vi "Convert String to Typed Value.vi"(8 "error in":errorcluster, 10 "Value":string, 11 "DataType":u16(ring) items=["UNKNOWN", "BOOLEAN", "INTEGER8", "INTEGER16", "INTEGER32", "UNSIGNED8", "UNSIGNED16", "UNSIGNED32", "REAL32", "VISIBLE_STRING", "OCTET_STRING", "UNICODE_STRING", "TIME_OF_DAY", "TIME_DIFFERENCE", "RESERVED1", "DOMAIN", "INTEGER24", "REAL64", "INTEGER40", "INTEGER48", "INTEGER56", "INTEGER64", "UNSIGNED24", "RESERVED2", "UNSIGNED40", "UNSIGNED48", "UNSIGNED56", "UNSIGNED64", "RESERVED3", "RESERVED4", "RESERVED5", "RESERVED6", "PDO_COMMUNICATION_PARAMETER", "PDO_MAPPING", "SDO_PARAMETER", "IDENTITY", "RESERVED7"]) -> (0 "error out":errorcluster, 3 "Typed Value":variant)   [LabVIEW 2020, in "CANopen.lvlib"]
uses:
  CANopen.lvlib
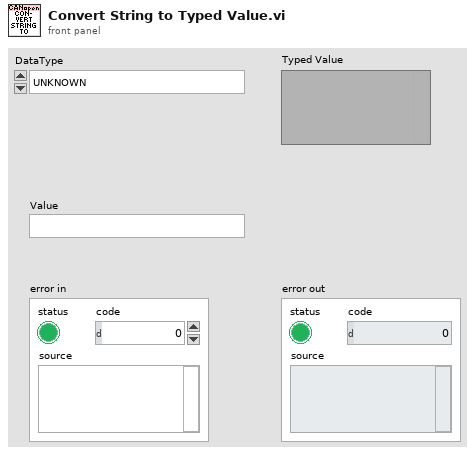
[diagram p1: front panel]
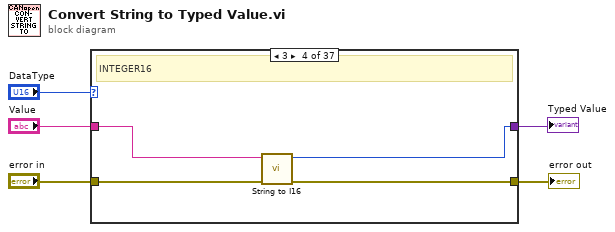
[diagram p0: block diagram]
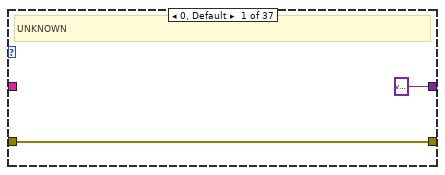
[diagram p2: hidden frame]
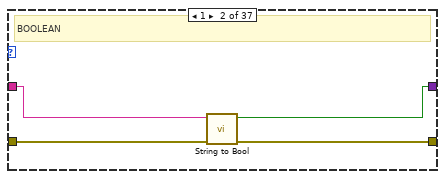
[diagram p3: hidden frame]
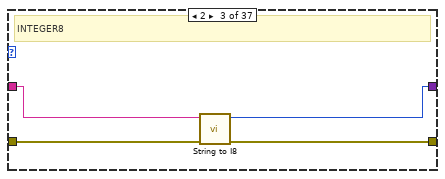
[diagram p4: hidden frame]
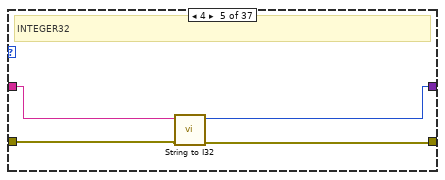
[diagram p5: hidden frame]
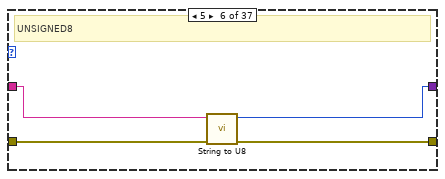
[diagram p6: hidden frame]
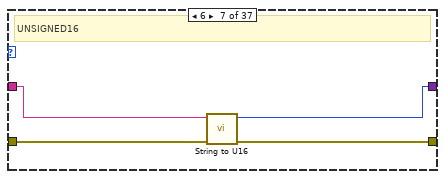
[diagram p7: hidden frame]
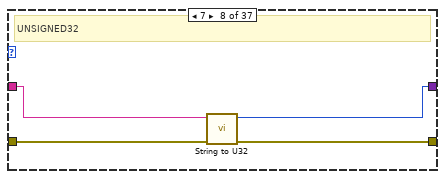
[diagram p8: hidden frame]
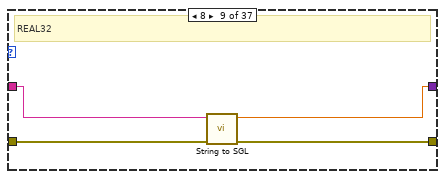
[diagram p9: hidden frame]
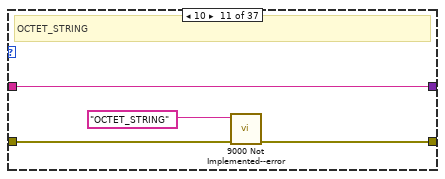
[diagram p11: hidden frame]
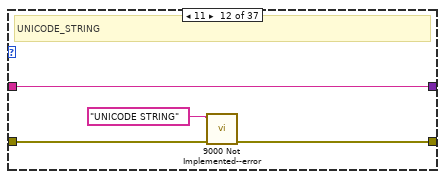
[diagram p12: hidden frame]
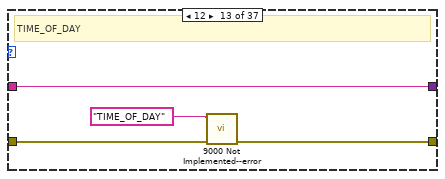
[diagram p13: hidden frame]
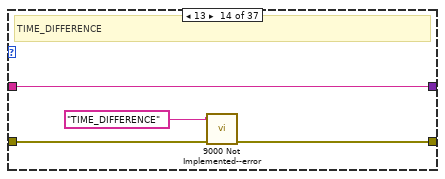
[diagram p14: hidden frame]
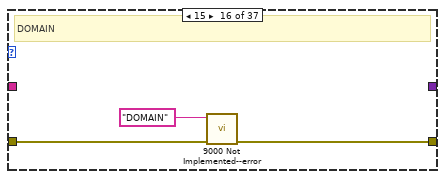
[diagram p16: hidden frame]
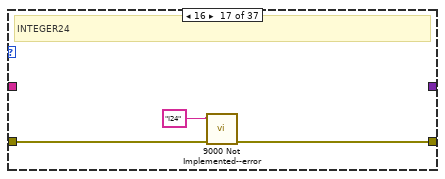
[diagram p17: hidden frame]
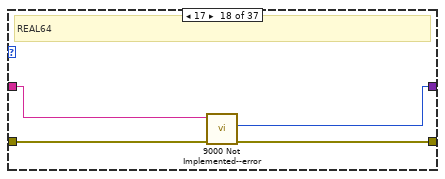
[diagram p18: hidden frame]
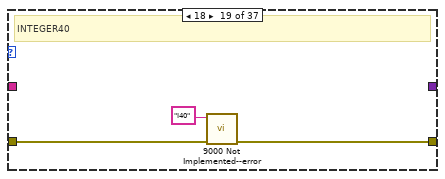
[diagram p19: hidden frame]
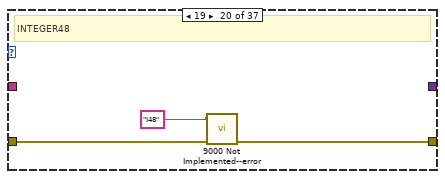
[diagram p20: hidden frame]
diagram:
  n1 = case shown="3" "DataType" {
    tunnel: [variant w8 w12 w16 w20 w24 w28 w32 w36 w41 w45 w48 w52 w57 _ _ _ w65 _ _ _ _ _ _ _ _ _ w94 _ _ _ _ _ _ _ _ _] -> w4
    tunnel: "error in" -> [w7 w11 w15 w19 w23 w27 w31 w35 w39 w40 w44 w49 w53 w56 w58 w61 w64 w68 w71 w74 w77 w80 w83 w84 w87 w90 w93 w97 w98 w99 w100 w101 w104 w107 w110 w113 w114]
    tunnel: [w7 w10 w13 w18 w22 w26 w30 w34 w38 w40 w43 w47 w51 w55 w58 w60 w63 w67 w70 w73 w76 w79 w82 w84 w86 w89 w92 w96 w98 w99 w100 w101 w103 w106 w109 w112 w114] -> w3
    tunnel: "Value" -> [_ w9 w14 w17 w21 w25 w29 w33 w37 w41 w45 w48 w52 w57 _ _ _ w66 _ _ _ w78 _ _ _ _ _ w95 _ _ _ _ _ _ _ _ _]
    frame 0, Default {
      # "UNKNOWN"
    }
    frame 1 {
      # "BOOLEAN"
      n2 = call "String to Bool.vi"("error in"=w11, "Integer String"=w9) -> ("error out"=w10:errorcluster, "Bool"=w8:bool)  [unwired: 8 in]
    }
    frame 2 {
      # "INTEGER8"
      n3 = call "String to I8.vi"("error in"=w15, "Integer String"=w14) -> ("error out"=w13:errorcluster, "I8"=w12:i8)  [unwired: 8 in]
    }
    frame 3 {
      # "INTEGER16"
      n4 = call "String to I16.vi"("error in"=w19, "Integer String"=w17) -> ("error out"=w18:errorcluster, "I16"=w16:i16)  [unwired: 8 in]
    }
    frame 4 {
      # "INTEGER32"
      n5 = call "String to I32.vi"("error in"=w23, "Integer String"=w21) -> ("error out"=w22:errorcluster, "I32"=w20:i32)  [unwired: 8 in]
    }
    frame 5 {
      # "UNSIGNED8"
      n6 = call "String to U8.vi"("error in"=w27, "Integer String"=w25) -> ("error out"=w26:errorcluster, "U8"=w24:u8)  [unwired: 8 in]
    }
    frame 6 {
      # "UNSIGNED16"
      n7 = call "String to U16.vi"("error in"=w31, "Integer String"=w29) -> ("error out"=w30:errorcluster, "U16"=w28:u16)  [unwired: 8 in]
    }
    frame 7 {
      # "UNSIGNED32"
      n8 = call "String to U32.vi"("error in"=w35, "Integer String"=w33) -> ("error out"=w34:errorcluster, "U32"=w32:u32)  [unwired: 8 in]
    }
    frame 8 {
      # "REAL32"
      n9 = call "String to SGL.vi"("error in"=w39, "Integer String"=w37) -> ("error out"=w38:errorcluster, "SGL"=w36:sgl)  [unwired: 8 in]
    }
    frame 9 {
      # "VISIBLE_STRING"
    }
    frame 10 {
      # "OCTET_STRING"
      n10 = call "9000 Not Implemented--error.vi"("error in"=w44, "Argument"="OCTET_STRING") -> ("error out"=w43:errorcluster)  [unwired: 8 in, 1 out]
    }
    frame 11 {
      # "UNICODE_STRING"
      n11 = call "9000 Not Implemented--error.vi"("error in"=w49, "Argument"="UNICODE STRING") -> ("error out"=w47:errorcluster)  [unwired: 8 in, 1 out]
    }
    frame 12 {
      # "TIME_OF_DAY"
      n12 = call "9000 Not Implemented--error.vi"("error in"=w53, "Argument"="TIME_OF_DAY") -> ("error out"=w51:errorcluster)  [unwired: 8 in, 1 out]
    }
    frame 13 {
      # "TIME_DIFFERENCE"
      n13 = call "9000 Not Implemented--error.vi"("error in"=w56, "Argument"="TIME_DIFFERENCE") -> ("error out"=w55:errorcluster)  [unwired: 8 in, 1 out]
    }
    frame 14 {
      # "RESERVED1"
    }
    frame 15 {
      # "DOMAIN"
      n14 = call "9000 Not Implemented--error.vi"("error in"=w61, "Argument"="DOMAIN") -> ("error out"=w60:errorcluster)  [unwired: 8 in, 1 out]
    }
    frame 16 {
      # "INTEGER24"
      n15 = call "9000 Not Implemented--error.vi"("error in"=w64, "Argument"="I24") -> ("error out"=w63:errorcluster)  [unwired: 8 in, 1 out]
    }
    frame 17 {
      # "REAL64"
      n16 = call "9000 Not Implemented--error.vi"("error in"=w68, "Argument"=w66) -> ("error out"=w67:errorcluster, "Error Code"=w65:i32)  [unwired: 8 in]
    }
    frame 18 {
      # "INTEGER40"
      n17 = call "9000 Not Implemented--error.vi"("error in"=w71, "Argument"="I40") -> ("error out"=w70:errorcluster)  [unwired: 8 in, 1 out]
    }
    frame 19 {
      # "INTEGER48"
      n18 = call "9000 Not Implemented--error.vi"("error in"=w74, "Argument"="I48") -> ("error out"=w73:errorcluster)  [unwired: 8 in, 1 out]
    }
    frame 20 {
      # "INTEGER56"
      n19 = call "9000 Not Implemented--error.vi"("error in"=w77, "Argument"="I56") -> ("error out"=w76:errorcluster)  [unwired: 8 in, 1 out]
    }
    frame 21 {
      # "INTEGER64"
      n20 = call "String to I64.vi"("error in"=w80, "Integer String"=w78) -> ("error out"=w79:errorcluster)  [unwired: 8 in, 1 out]
    }
    frame 22 {
      # "UNSIGNED24"
      n21 = call "9000 Not Implemented--error.vi"("error in"=w83, "Argument"="U24") -> ("error out"=w82:errorcluster)  [unwired: 8 in, 1 out]
    }
    frame 23 {
      # "RESERVED2"
    }
    frame 24 {
      # "UNSIGNED40"
      n22 = call "9000 Not Implemented--error.vi"("error in"=w87, "Argument"="U40") -> ("error out"=w86:errorcluster)  [unwired: 8 in, 1 out]
    }
    frame 25 {
      # "UNSIGNED48"
      n23 = call "9000 Not Implemented--error.vi"("error in"=w90, "Argument"="U48") -> ("error out"=w89:errorcluster)  [unwired: 8 in, 1 out]
    }
    frame 26 {
      # "UNSIGNED56"
      n24 = call "9000 Not Implemented--error.vi"("error in"=w93, "Argument"="U56") -> ("error out"=w92:errorcluster)  [unwired: 8 in, 1 out]
    }
    frame 27 {
      # "UNSIGNED64"
      n25 = call "String to U64.vi"("error in"=w97, "Integer String"=w95) -> ("error out"=w96:errorcluster, "U64"=w94:u64)  [unwired: 8 in]
    }
    frame 28 {
      # "RESERVED3"
    }
    frame 29 {
      # "RESERVED4"
    }
    frame 30 {
      # "RESERVED5"
    }
    frame 31 {
      # "RESERVED6"
    }
    frame 32 {
      # "PDO_COMMUNICATION_PARAMETER"
      n26 = call "9000 Not Implemented--error.vi"("error in"=w104, "Argument"="PDO_COMMUNICATION_PARAMETER") -> ("error out"=w103:errorcluster)  [unwired: 8 in, 1 out]
    }
    frame 33 {
      # "PDO_MAPPING"
      n27 = call "9000 Not Implemented--error.vi"("error in"=w107, "Argument"="PDO_MAPPING") -> ("error out"=w106:errorcluster)  [unwired: 8 in, 1 out]
    }
    frame 34 {
      # "SDO_PARAMETER"
      n28 = call "9000 Not Implemented--error.vi"("error in"=w110, "Argument"="SDO_PARAMETER") -> ("error out"=w109:errorcluster)  [unwired: 8 in, 1 out]
    }
    frame 35 {
      # "IDENTITY"
      n29 = call "9000 Not Implemented--error.vi"("error in"=w113, "Argument"="IDENTITY") -> ("error out"=w112:errorcluster)  [unwired: 8 in, 1 out]
    }
    frame 36 {
      # "RESERVED7"
    }
  }
  "Typed Value" <- w4
  "error out" <- w3
